vi "Write Document Bounds.vi"(5 "Document Bounds":T1, 9 "Text in":refnum<class "Text.lvclass">) -> (3 "Text out":refnum<class "Text.lvclass">)   [LabVIEW 2014, in "Text.lvclass"]
uses:
  Text.lvclass
  <vilib>/Utility/miscctls.llb/LVBoundsTypeDef.ctl
  Text.lvclass/Text.ctl
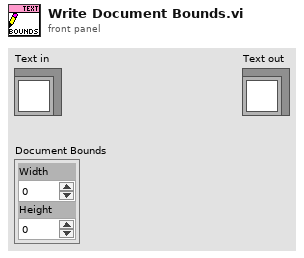
[diagram p1: front panel]
types:
  T1 = typedef "LVBoundsTypeDef.ctl" = cluster{"Width":u32, "Height":u32}
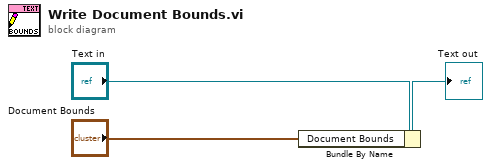
[diagram p0: block diagram]
diagram:
  n1 = Bundle By Name(cluster="Text in", "Document Bounds"="Document Bounds") -> (→"Text out":refnum<class "Text.lvclass">)
